vi "asynch_wait_example_1.vi"() -> ()   [LabVIEW 2015]
uses:
  polys/poly_asynch_wait_start.vi
  polys/poly_asynch_wait_notify.vi
  polys/poly_asynch_wait_stop.vi
  polys/poly_asynch_wait_wait.vi
panel:
  out "4 wait time":u32
  out "3 wait time":u32
  out "2 wait time":u32
  out "1 wait time":u32
  in  "stop":bool
  out "4 refnum":u32
  out "3 refnum":u32
  out "2 refnum":u32
  out "1 refnum":u32
  in  "4 stop":bool
  in  "3 stop":bool
  in  "2 stop":bool
  in  "4 notify":bool
  in  "3 notify":bool
  in  "2 notify":bool
  in  "4 timeout":i32=-1 format="%.0f ms"
  in  "3 timeout":i32=3000 format="%.0f ms"
  in  "2 timeout":i32=2000 format="%.0f ms"
  in  "1 timeout":i32=1000 format="%.0f ms"
  in  "1 stop":bool
  in  "1 notify":bool
  out "4 error":bool
  out "3 error":bool
  out "2 error":bool
  out "1 error":bool
  out "4 timeout":bool
  out "3 timeout":bool
  out "2 timeout":bool
  out "1 tiemout":bool
  out "4 done":bool
  out "3 done":bool
  out "2 done":bool
  out "1 done":bool
  # "notifier refnum"
  # "timeout [ms]"
  # "done"
  # "timed out"
  # "error"
  # "send notif."
  # "send notif."
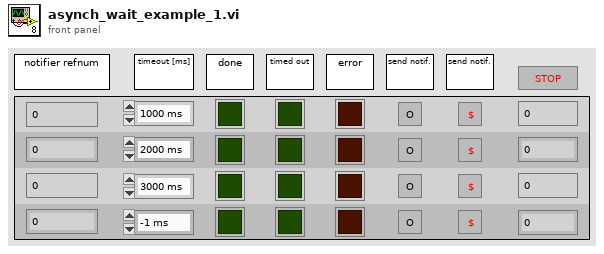
[diagram p1: front panel]
types:
  T1 = typedef "boolean_notifier.ctl" = refnum<notifier>
  T2 = typedef "asynch_wait_ref.ctl" = cluster{"vi ref":refnum<vi>, "TF notifier":T1}
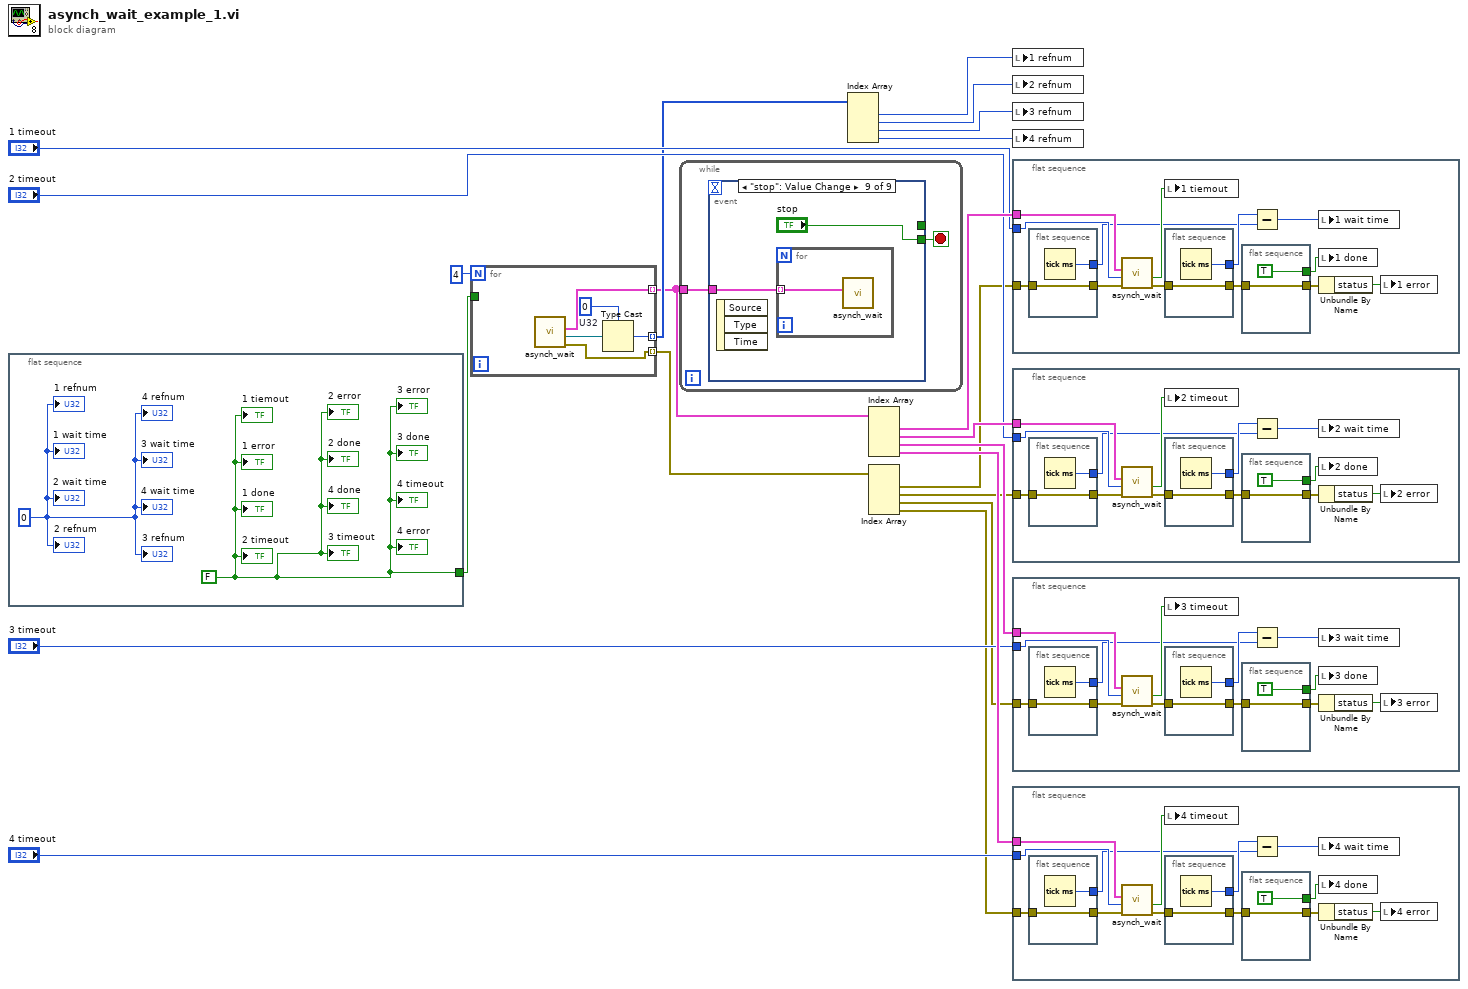
[diagram p0: block diagram]
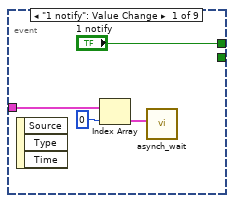
[diagram p2: hidden frame]
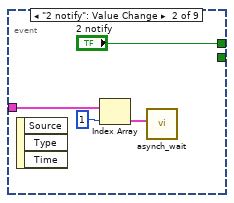
[diagram p3: hidden frame]
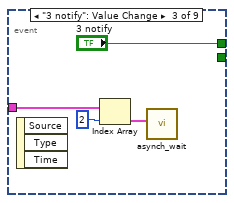
[diagram p4: hidden frame]
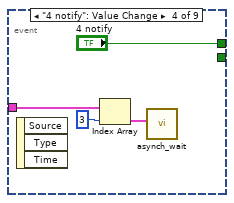
[diagram p5: hidden frame]
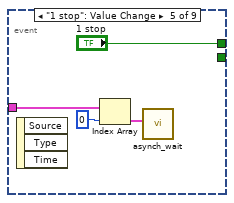
[diagram p6: hidden frame]
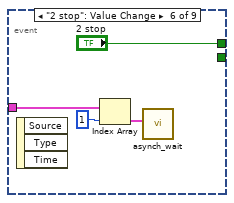
[diagram p7: hidden frame]
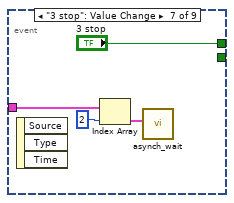
[diagram p8: hidden frame]
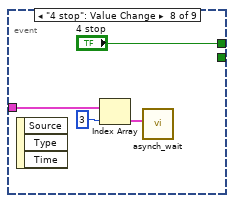
[diagram p9: hidden frame]
diagram:
  n1 = flat-sequence {
    tunnel: [w22] -> w17
    frame #0 {
      w22 = FALSE
      w23 = u32 0
      "1 done" <- w22
      "2 done" <- w22
      "3 done" <- w22
      "4 done" <- w22
      "1 tiemout" <- w22
      "2 timeout" <- w22
      "3 timeout" <- w22
      "4 timeout" <- w22
      "1 error" <- w22
      "2 error" <- w22
      "3 error" <- w22
      "4 error" <- w22
      "1 refnum" <- w23
      "2 refnum" <- w23
      "3 refnum" <- w23
      "4 refnum" <- w23
      "1 wait time" <- w23
      "2 wait time" <- w23
      "3 wait time" <- w23
      "4 wait time" <- w23
    }
  }
  n2 = for {
    N: 4 -> [_]
    tunnel: [w27] -> w11 mode=indexing
    tunnel: [w25] -> w10 mode=indexing
    tunnel: w17 -> [_]
    tunnel: [w24] -> w5 mode=indexing
    w28 = u32 0  # U32
    n3 = call-poly "asynch_wait.vi"() -> ("error out"=w24:errorcluster, "notifier"=w26:T1, "asynch wait ref out"=w25:T2)  [unwired: 9 in]
    n4 = Type Cast(type=w28, x=w26) -> (*(type *) &x=w27:u32)
  }
  n5 = while {
    tunnel: w10 -> [w30]
    stop <- w29 stop-if-true
    n6 = event shown="[8] \"stop\": Value Change" {
      selector: _ -> [_ _ _ _ _ _ _ _ _]
      dyn-events: _ -> [_ _ _ _ _ _ _ _ _]
      timeout: _ -> [_ _ _ _ _ _ _ _ _]
      tunnel: w30 -> [w34 w38 w42 w46 w50 w54 w58 w62 w63]
      tunnel: ["1 notify" "2 notify" "3 notify" "4 notify" "1 stop" "2 stop" "3 stop" "4 stop" _] -> _
      tunnel: [_ _ _ _ _ _ _ _ "stop"] -> w29
      event "1 notify": Value Change {
        n7 = event-data() -> ()  [unwired: 1 in, 3 out]
        n8 = Index Array(array=w34, index=0) -> (element=w31:T2)
        n9 = call-poly "asynch_wait.vi"("asynch wait ref in"=w31) -> ()  [unwired: 10 in, 1 out]
      }
      event "2 notify": Value Change {
        n10 = event-data() -> ()  [unwired: 1 in, 3 out]
        n11 = Index Array(array=w38, index=1) -> (element=w35:T2)
        n12 = call-poly "asynch_wait.vi"("asynch wait ref in"=w35) -> ()  [unwired: 10 in, 1 out]
      }
      event "3 notify": Value Change {
        n13 = event-data() -> ()  [unwired: 1 in, 3 out]
        n14 = Index Array(array=w42, index=2) -> (element=w39:T2)
        n15 = call-poly "asynch_wait.vi"("asynch wait ref in"=w39) -> ()  [unwired: 10 in, 1 out]
      }
      event "4 notify": Value Change {
        n16 = event-data() -> ()  [unwired: 1 in, 3 out]
        n17 = Index Array(array=w46, index=3) -> (element=w43:T2)
        n18 = call-poly "asynch_wait.vi"("asynch wait ref in"=w43) -> ()  [unwired: 10 in, 1 out]
      }
      event "1 stop": Value Change {
        n19 = event-data() -> ()  [unwired: 1 in, 3 out]
        n20 = Index Array(array=w50, index=0) -> (element=w48:T2)
        n21 = call-poly "asynch_wait.vi"("asynch wait ref in"=w48) -> ()  [unwired: 9 in, 2 out]
      }
      event "2 stop": Value Change {
        n22 = event-data() -> ()  [unwired: 1 in, 3 out]
        n23 = Index Array(array=w54, index=1) -> (element=w52:T2)
        n24 = call-poly "asynch_wait.vi"("asynch wait ref in"=w52) -> ()  [unwired: 9 in, 2 out]
      }
      event "3 stop": Value Change {
        n25 = event-data() -> ()  [unwired: 1 in, 3 out]
        n26 = Index Array(array=w58, index=2) -> (element=w56:T2)
        n27 = call-poly "asynch_wait.vi"("asynch wait ref in"=w56) -> ()  [unwired: 9 in, 2 out]
      }
      event "4 stop": Value Change {
        n28 = event-data() -> ()  [unwired: 1 in, 3 out]
        n29 = Index Array(array=w62, index=3) -> (element=w60:T2)
        n30 = call-poly "asynch_wait.vi"("asynch wait ref in"=w60) -> ()  [unwired: 9 in, 2 out]
      }
      event "stop": Value Change {
        n31 = event-data() -> ()  [unwired: 1 in, 3 out]
        n32 = for {
          tunnel: w63 -> [w65] mode=indexing
          n33 = call-poly "asynch_wait.vi"("asynch wait ref in"=w65) -> ()  [unwired: 9 in, 2 out]
        }
      }
    }
  }
  n34 = Index Array(array=w11) -> (element #1=w9:u32, element #2=w6:u32, element #3=w8:u32, element #4=w7:u32)  [unwired: 4 in]
  n35 = Index Array(array=w10) -> (element #1=w20:T2, element #2=w19:T2, element #3=w18:T2, element #4=w16:T2)  [unwired: 4 in]
  n36 = Index Array(array=w5) -> (element #1=w4:errorcluster, element #2=w3:errorcluster, element #3=w2:errorcluster, element #4=w1:errorcluster)  [unwired: 4 in]
  n37 = local write "1 refnum"(w9) -> ()
  n38 = local write "2 refnum"(w6) -> ()
  n39 = local write "3 refnum"(w8) -> ()
  n40 = local write "4 refnum"(w7) -> ()
  n41 = flat-sequence {
    tunnel: w20 -> [w78]
    tunnel: "1 timeout" -> [w75]
    tunnel: w4 -> [w71]
    frame #0 {
      n42 = flat-sequence {
        tunnel: [w82] -> w67
        tunnel: [w81] -> w72
        tunnel: w71 -> [w81]
        frame #0 {
          n43 = Tick Count (ms)() -> (millisecond timer value=w82:u32)
        }
      }
      n44 = call-poly "asynch_wait.vi"("error in"=w72, "timeout [ms]"=w75, "asynch wait ref in"=w78) -> ("error out"=w70:errorcluster, "timed out?"=w77:bool)  [unwired: 5 in, 2 out]
      n45 = local write "1 tiemout"(w77) -> ()
      n46 = flat-sequence {
        tunnel: [w80] -> w68
        tunnel: [w79] -> w69
        tunnel: w70 -> [w79]
        frame #0 {
          n47 = Tick Count (ms)() -> (millisecond timer value=w80:u32)
        }
      }
      n48 = flat-sequence {
        tunnel: [TRUE] -> w73
        tunnel: [w83] -> w74
        tunnel: w69 -> [w83]
        frame #0 {
        }
      }
      n49 = Subtract(x=w68, y=w67) -> (x-y=w66:u32)
      n50 = local write "1 wait time"(w66) -> ()
      n51 = local write "1 done"(w73) -> ()
      n52 = Unbundle By Name(w74) -> ("status"=w76:bool)
      n53 = local write "1 error"(w76) -> ()
    }
  }
  n54 = flat-sequence {
    tunnel: w19 -> [w97]
    tunnel: "2 timeout" -> [w94]
    tunnel: w3 -> [w91]
    frame #0 {
      n55 = flat-sequence {
        tunnel: [w101] -> w86
        tunnel: [w100] -> w90
        tunnel: w91 -> [w100]
        frame #0 {
          n56 = Tick Count (ms)() -> (millisecond timer value=w101:u32)
        }
      }
      n57 = call-poly "asynch_wait.vi"("error in"=w90, "timeout [ms]"=w94, "asynch wait ref in"=w97) -> ("error out"=w89:errorcluster, "timed out?"=w96:bool)  [unwired: 5 in, 2 out]
      n58 = local write "2 timeout"(w96) -> ()
      n59 = flat-sequence {
        tunnel: [w99] -> w87
        tunnel: [w98] -> w88
        tunnel: w89 -> [w98]
        frame #0 {
          n60 = Tick Count (ms)() -> (millisecond timer value=w99:u32)
        }
      }
      n61 = flat-sequence {
        tunnel: [TRUE] -> w92
        tunnel: [w102] -> w93
        tunnel: w88 -> [w102]
        frame #0 {
        }
      }
      n62 = Subtract(x=w87, y=w86) -> (x-y=w85:u32)
      n63 = local write "2 wait time"(w85) -> ()
      n64 = local write "2 done"(w92) -> ()
      n65 = Unbundle By Name(w93) -> ("status"=w95:bool)
      n66 = local write "2 error"(w95) -> ()
    }
  }
  n67 = flat-sequence {
    tunnel: w18 -> [w116]
    tunnel: "3 timeout" -> [w113]
    tunnel: w2 -> [w110]
    frame #0 {
      n68 = flat-sequence {
        tunnel: [w120] -> w105
        tunnel: [w119] -> w109
        tunnel: w110 -> [w119]
        frame #0 {
          n69 = Tick Count (ms)() -> (millisecond timer value=w120:u32)
        }
      }
      n70 = call-poly "asynch_wait.vi"("error in"=w109, "timeout [ms]"=w113, "asynch wait ref in"=w116) -> ("error out"=w108:errorcluster, "timed out?"=w115:bool)  [unwired: 5 in, 2 out]
      n71 = local write "3 timeout"(w115) -> ()
      n72 = flat-sequence {
        tunnel: [w118] -> w106
        tunnel: [w117] -> w107
        tunnel: w108 -> [w117]
        frame #0 {
          n73 = Tick Count (ms)() -> (millisecond timer value=w118:u32)
        }
      }
      n74 = flat-sequence {
        tunnel: [TRUE] -> w111
        tunnel: [w121] -> w112
        tunnel: w107 -> [w121]
        frame #0 {
        }
      }
      n75 = Subtract(x=w106, y=w105) -> (x-y=w104:u32)
      n76 = local write "3 wait time"(w104) -> ()
      n77 = local write "3 done"(w111) -> ()
      n78 = Unbundle By Name(w112) -> ("status"=w114:bool)
      n79 = local write "3 error"(w114) -> ()
    }
  }
  n80 = flat-sequence {
    tunnel: w16 -> [w132]
    tunnel: "4 timeout" -> [w131]
    tunnel: w1 -> [w129]
    frame #0 {
      n81 = flat-sequence {
        tunnel: [w139] -> w124
        tunnel: [w138] -> w128
        tunnel: w129 -> [w138]
        frame #0 {
          n82 = Tick Count (ms)() -> (millisecond timer value=w139:u32)
        }
      }
      n83 = call-poly "asynch_wait.vi"("error in"=w128, "timeout [ms]"=w131, "asynch wait ref in"=w132) -> ("error out"=w127:errorcluster, "timed out?"=w134:bool)  [unwired: 5 in, 2 out]
      n84 = local write "4 timeout"(w134) -> ()
      n85 = flat-sequence {
        tunnel: [w137] -> w125
        tunnel: [w136] -> w126
        tunnel: w127 -> [w136]
        frame #0 {
          n86 = Tick Count (ms)() -> (millisecond timer value=w137:u32)
        }
      }
      n87 = flat-sequence {
        tunnel: [TRUE] -> w135
        tunnel: [w140] -> w130
        tunnel: w126 -> [w140]
        frame #0 {
        }
      }
      n88 = Subtract(x=w125, y=w124) -> (x-y=w123:u32)
      n89 = local write "4 wait time"(w123) -> ()
      n90 = local write "4 done"(w135) -> ()
      n91 = Unbundle By Name(w130) -> ("status"=w133:bool)
      n92 = local write "4 error"(w133) -> ()
    }
  }
